vi "I2C Read Data.vi"(5 "Address":T1 format="%02x", 6 "NoStop (F)":bool, 7 "I2C #":T2=-1, 8 "error in (no error)":errorcluster, 9 "Len":u8, 11 "DeviceComms in":refnum<class "DeviceComms.lvclass">) -> (0 "error out":errorcluster, 1 "Data":string, 3 "DeviceComms out":refnum<class "DeviceComms.lvclass">)   [LabVIEW 2020, in "CTI.lvlib" / "DeviceComms.lvclass"]
uses:
  DeviceComms.lvclass
  I2C Number.ctl
  CTI.lvlib
  I2C Address.ctl
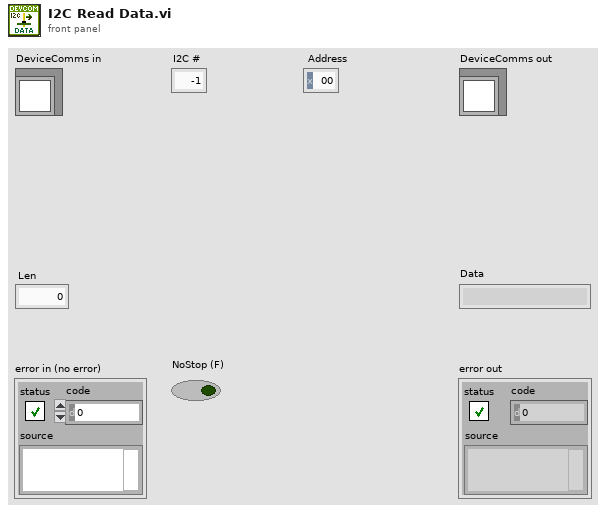
[diagram p1: front panel]
types:
  T1 = typedef "CTI.lvlib/I2C Address.ctl" = u8
  T2 = typedef "CTI.lvlib/I2C Number.ctl" = i8
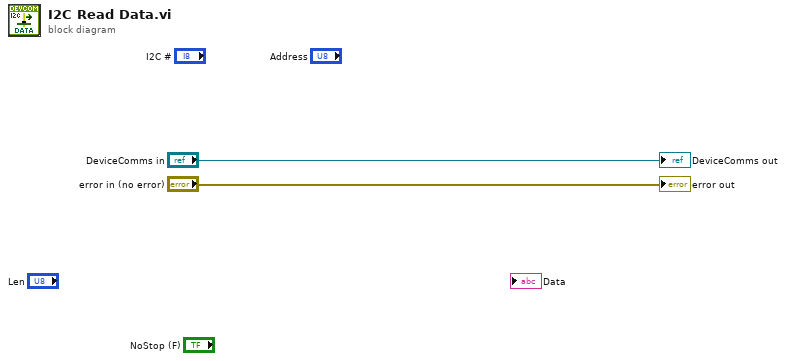
[diagram p0: block diagram]
diagram:
  "error out" <- "error in (no error)"
  "DeviceComms out" <- "DeviceComms in"
